vi "Feedback Evaporative Cooler Demo.vi"() -> ()   [LabVIEW 2012]
uses:
  Cooler UI/Cooler Panel/Cooler Panel.lvclass
  Cooler/Cooler/Cooler.lvclass
  <vilib>/ActorFramework/Message Queue/Message Queue.lvclass/Message Queue.ctl
  Cooler/Cooler Messages/Write UI Msg/Write UI Msg.lvclass/Write UI Msg.ctl
  <vilib>/ActorFramework/Message Enqueuer/Message Enqueuer.lvclass/Message Enqueuer.ctl
  Cooler UI/Cooler UI with Events Messages/Write Cooler Msg/Write Cooler Msg.lvclass/Write Cooler Msg.ctl
  <vilib>/ActorFramework/Message Enqueuer/Enqueue.vi
  <vilib>/ActorFramework/Message Priority Queue/Priority Enqueue.vi
  Cooler/Cooler Messages/Write UI Msg/Write UI Msg.lvclass
  Cooler UI/Cooler UI with Events Messages/Write Cooler Msg/Write Cooler Msg.lvclass
  <vilib>/ActorFramework/Stop Msg/Stop Msg.lvclass
  <vilib>/ActorFramework/Actor/Actor.lvclass
  <vilib>/ActorFramework/Message Queue/Message Queue.lvclass
panel:
  in  "Stop Button":bool
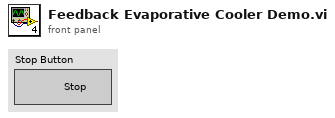
[diagram p1: front panel]
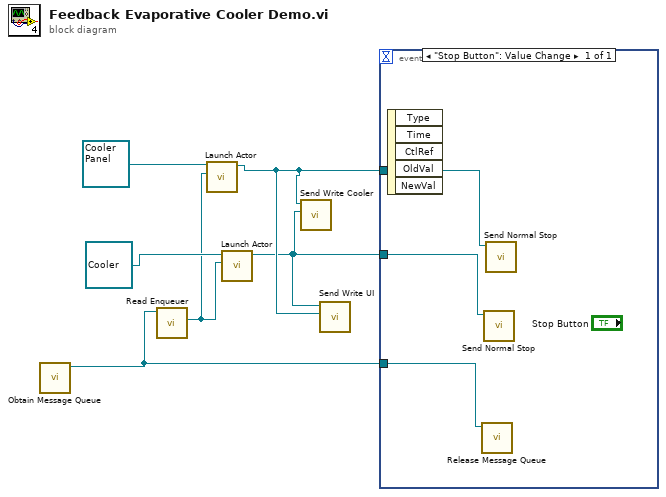
[diagram p0: block diagram]
diagram:
  n1 = call <vilib>:"Obtain Message Queue.vi"() -> ("Message Queue"=w3:refnum<class "Message Queue.lvclass">)  [unwired: 10 in, 1 out]
  n2 = call <vilib>:"Read Enqueuer.vi"("Message Queue"=w3) -> ("Message Enqueuer"=w4:refnum<class "Message Enqueuer.lvclass">)  [unwired: 10 in]
  n3 = call <vilib>:"Launch Actor.vi"("Actor-to-Caller Enqueuer"=w4, "Actor"=refnum<class "Cooler Panel.lvclass"> refnum ("Cooler UI.lvlib:Cooler Panel.lvclass")) -> ("Caller-To-Actor Enqueuer"=w2:refnum<class "Message Enqueuer.lvclass">)  [unwired: 8 in, 1 out]
  n4 = call <vilib>:"Launch Actor.vi"("Actor-to-Caller Enqueuer"=w4, "Actor"=refnum<class "Cooler.lvclass"> refnum ("Cooler.lvlib:Cooler.lvclass")) -> ("Caller-To-Actor Enqueuer"=w1:refnum<class "Message Enqueuer.lvclass">)  [unwired: 8 in, 1 out]
  n5 = call "Send Write Cooler.vi"("Cooler"=w1, "Message Enqueuer"=w2) -> ()  [unwired: 8 in, 2 out]
  n6 = call "Send Write UI.vi"("UI"=w2, "Message Enqueuer"=w1) -> ()  [unwired: 8 in, 2 out]
  n7 = event shown="[0] \"Stop Button\": Value Change" {
    selector: _ -> [_]
    dyn-events: _ -> [_]
    timeout: _ -> [_]
    tunnel: w3 -> [w9]
    tunnel: w1 -> [w7]
    tunnel: w2 -> [w8]
    event "Stop Button": Value Change {
      n8 = event-data() -> ()  [unwired: 1 in, 5 out]
      n9 = call <vilib>:"Release Message Queue.vi"("Message Queue"=w9) -> ()  [unwired: 9 in, 2 out]
      n10 = call <vilib>:"Send Normal Stop.vi"("Message Enqueuer"=w7) -> ()  [unwired: 10 in, 1 out]
      n11 = call <vilib>:"Send Normal Stop.vi"("Message Enqueuer"=w8) -> ()  [unwired: 10 in, 1 out]
    }
  }
